vi "DC filter(Sub VI).vi"(0 "AI0 input":dbl[](array[numeric]), 1 "AI1 input":dbl[](array[numeric]), 2 "AI2 input":dbl[](array[numeric]), 3 "AI3 input":dbl[](array[numeric]), 4 "AI4 input":dbl[](array[numeric]), 5 "AI5 input":dbl[](array[numeric]), 6 "AI6 input":dbl[](array[numeric]), 7 "AI7 input":dbl[](array[numeric]), 8 "sum input (回授)":dbl[](array[numeric]), 9 "DAQ AI":dbl[](array[numeric]), 10 "迴圈數":i32, 11 "ÂoDC°}¦C¤j¤p":i32) -> (17 "sum out":dbl[](array[numeric]), 18 "DC Filter out":dbl[](array[numeric]), 19 "DC value":dbl[](array[numeric]), 20 "AI0 output":dbl[](array[numeric]), 21 "AI1 output":dbl[](array[numeric]), 22 "AI2 output":dbl[](array[numeric]), 23 "AI3 output":dbl[](array[numeric]), 24 "AI4 output":dbl[](array[numeric]), 25 "AI5 output":dbl[](array[numeric]), 26 "AI6 output":dbl[](array[numeric]), 27 "AI7 output":dbl[](array[numeric]))   [LabVIEW 2010]
panel:
  # "output"
  # "input"
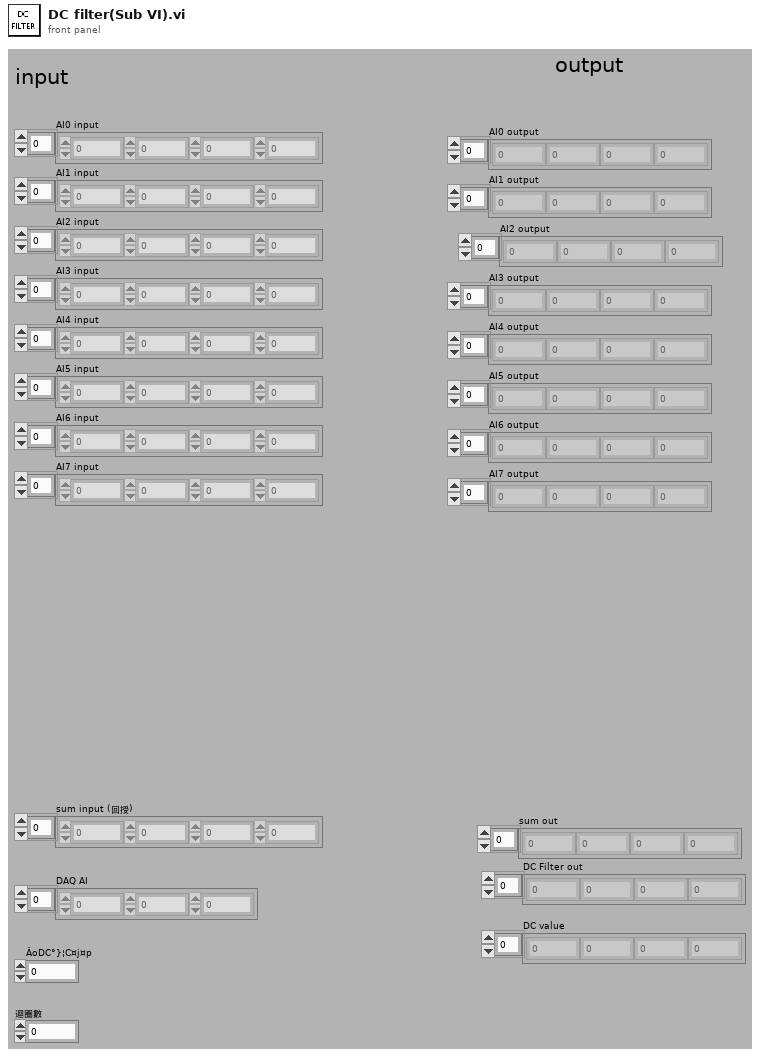
[diagram p1: front panel]
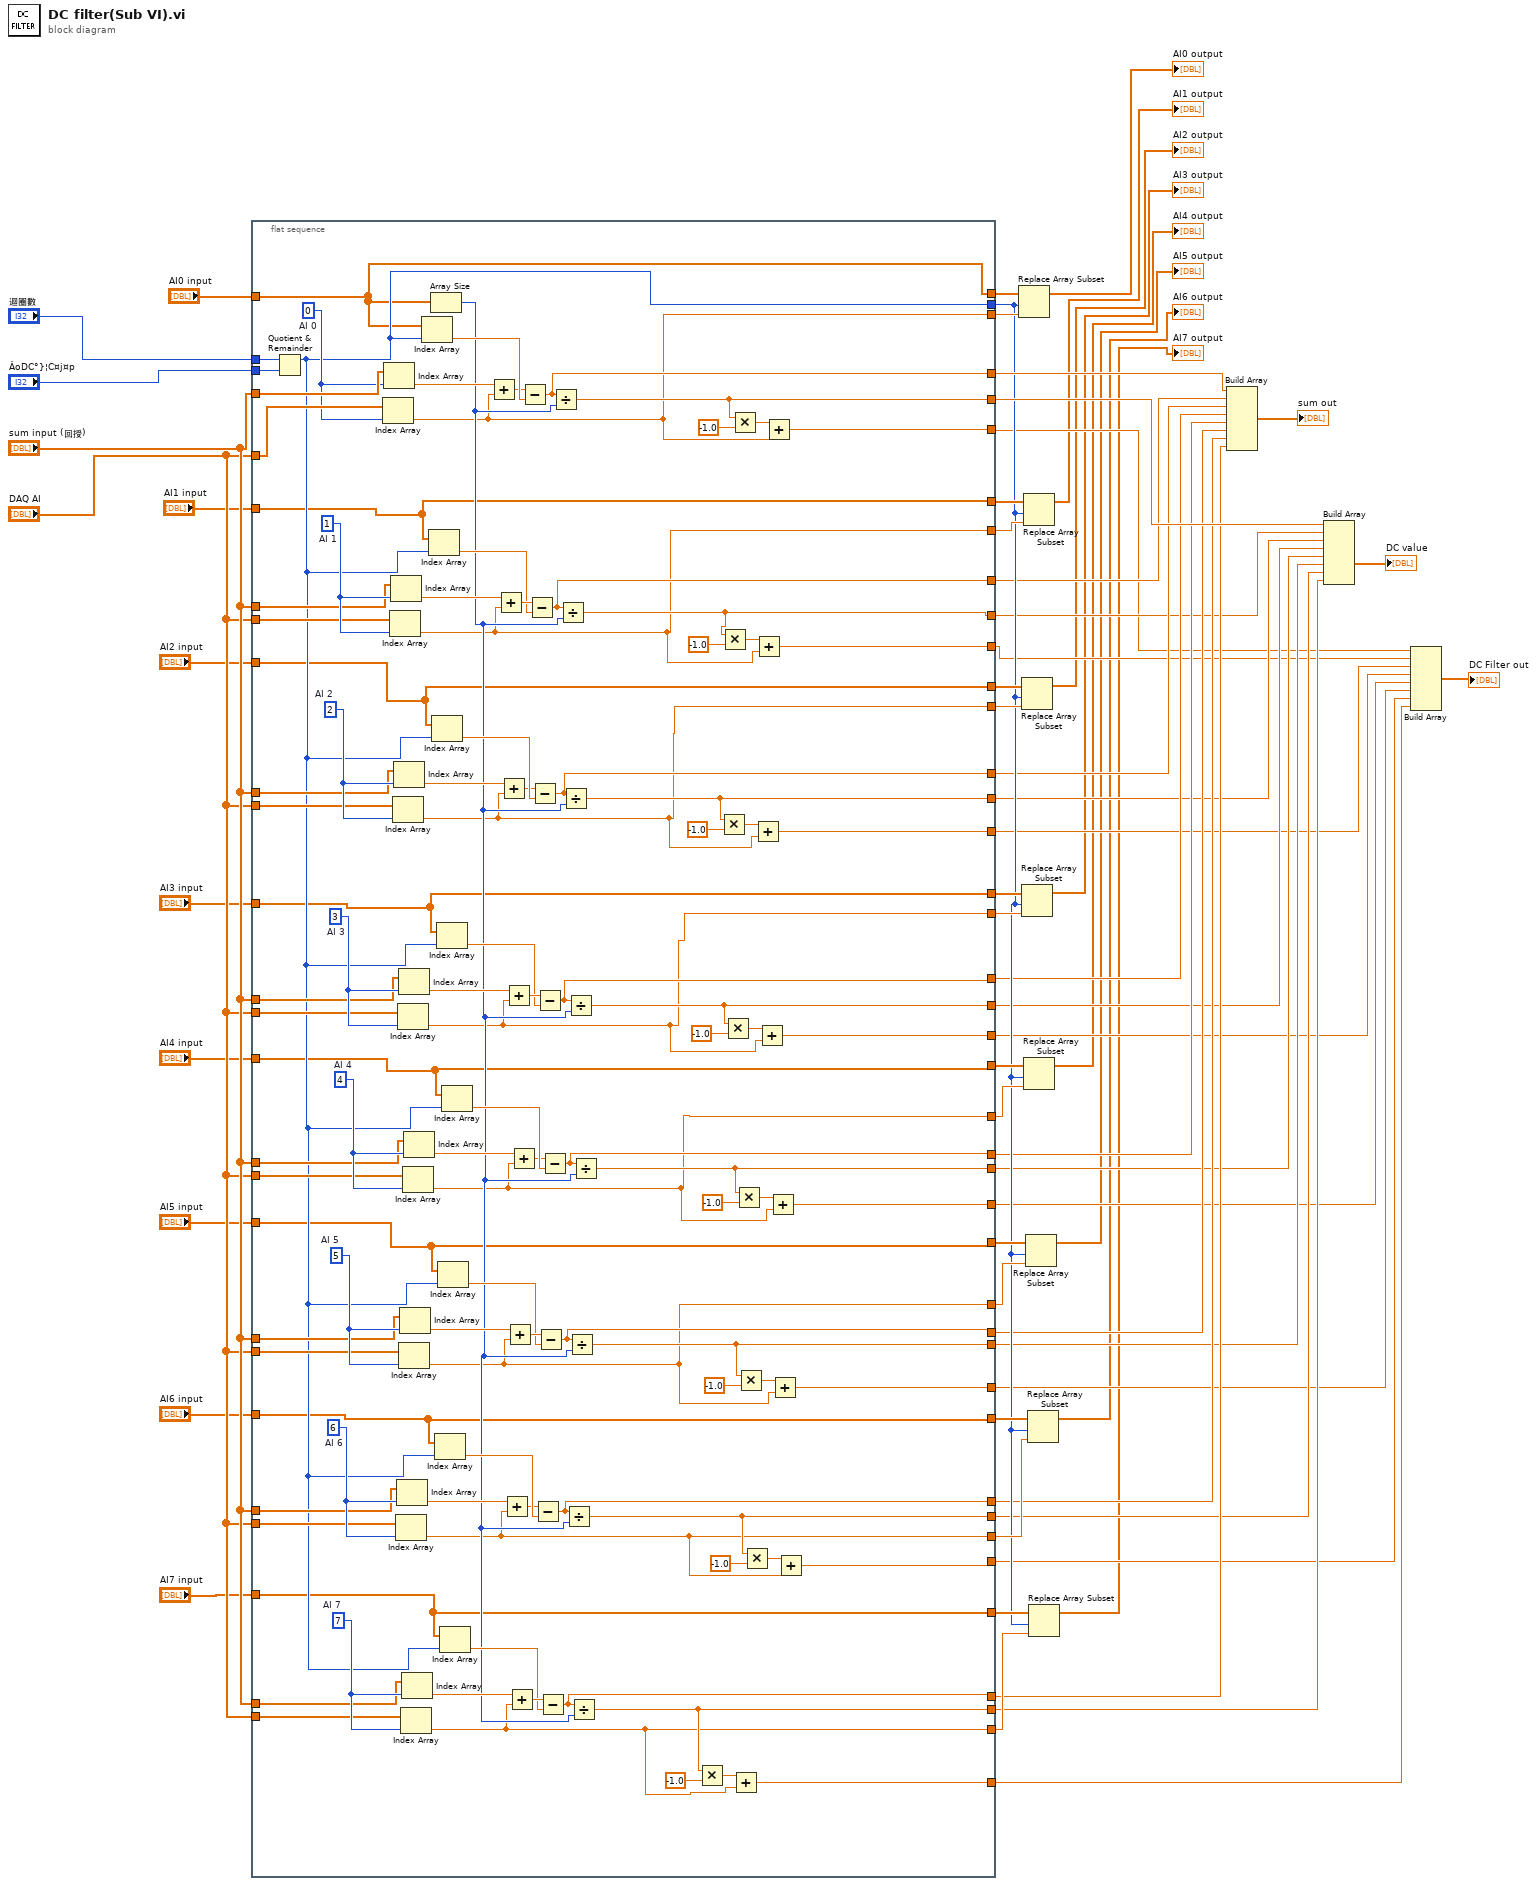
[diagram p0: block diagram]
diagram:
  n1 = flat-sequence {
    tunnel: [w109] -> w62
    tunnel: [w121] -> w42
    tunnel: [w72] -> w61
    tunnel: "迴圈數" -> [w164]
    tunnel: "sum input (回授)" -> [w169]
    tunnel: "DAQ AI" -> [w168]
    tunnel: "ÂoDC°}¦C¤j¤p" -> [w167]
    tunnel: [w112] -> w60
    tunnel: [w165] -> w63
    tunnel: "sum input (回授)" -> [w159]
    tunnel: "DAQ AI" -> [w158]
    tunnel: [w71] -> w57
    tunnel: [w105] -> w56
    tunnel: "sum input (回授)" -> [w153]
    tunnel: "DAQ AI" -> [w152]
    tunnel: [w70] -> w55
    tunnel: [w101] -> w54
    tunnel: "sum input (回授)" -> [w147]
    tunnel: "DAQ AI" -> [w146]
    tunnel: [w69] -> w53
    tunnel: [w97] -> w52
    tunnel: "sum input (回授)" -> [w129]
    tunnel: "sum input (回授)" -> [w128]
    tunnel: "sum input (回授)" -> [w127]
    tunnel: "sum input (回授)" -> [w126]
    tunnel: "DAQ AI" -> [w125]
    tunnel: "DAQ AI" -> [w124]
    tunnel: "DAQ AI" -> [w123]
    tunnel: "DAQ AI" -> [w122]
    tunnel: [w68] -> w49
    tunnel: [w93] -> w48
    tunnel: [w67] -> w47
    tunnel: [w89] -> w46
    tunnel: [w66] -> w45
    tunnel: [w85] -> w44
    tunnel: [w65] -> w43
    tunnel: [w81] -> w40
    tunnel: [w120] -> w39
    tunnel: [w119] -> w38
    tunnel: [w118] -> w37
    tunnel: [w117] -> w36
    tunnel: [w116] -> w35
    tunnel: [w115] -> w34
    tunnel: [w114] -> w33
    tunnel: [w106] -> w32
    tunnel: [w102] -> w31
    tunnel: [w98] -> w30
    tunnel: [w94] -> w29
    tunnel: [w90] -> w28
    tunnel: [w86] -> w27
    tunnel: [w82] -> w26
    tunnel: [w80] -> w17
    tunnel: [w79] -> w18
    tunnel: [w78] -> w19
    tunnel: [w77] -> w20
    tunnel: [w76] -> w21
    tunnel: [w75] -> w22
    tunnel: [w74] -> w23
    tunnel: [w73] -> w24
    tunnel: "AI0 input" -> [w72]
    tunnel: "AI1 input" -> [w71]
    tunnel: "AI2 input" -> [w70]
    tunnel: "AI3 input" -> [w69]
    tunnel: "AI4 input" -> [w68]
    tunnel: "AI5 input" -> [w67]
    tunnel: "AI6 input" -> [w66]
    tunnel: "AI7 input" -> [w65]
    frame #0 {
      w133 = 7  # AI 7
      w134 = 6  # AI 6
      w141 = 5  # AI 5
      w142 = 4  # AI 4
      w151 = 3  # AI 3
      w154 = 2  # AI 2
      w163 = 1  # AI 1
      w166 = 0  # AI 0
      n2 = Quotient & Remainder(x=w164, y=w167) -> (x-y*floor(x/y)=w121:i32)  [unwired: 1 out]
      n3 = Index Array(array=w168, index=w166) -> (element=w109:dbl)
      n4 = Index Array(array=w169, index=w166) -> (element=w170:dbl)
      n5 = Index Array(array=w158, index=w163) -> (element=w105:dbl)
      n6 = Index Array(array=w159, index=w163) -> (element=w162:dbl)
      n7 = Index Array(array=w152, index=w154) -> (element=w101:dbl)
      n8 = Index Array(array=w153, index=w154) -> (element=w155:dbl)
      n9 = Index Array(array=w123, index=w134) -> (element=w85:dbl)
      n10 = Index Array(array=w127, index=w134) -> (element=w135:dbl)
      n11 = Index Array(array=w146, index=w151) -> (element=w97:dbl)
      n12 = Index Array(array=w147, index=w151) -> (element=w150:dbl)
      n13 = Index Array(array=w124, index=w141) -> (element=w89:dbl)
      n14 = Index Array(array=w128, index=w141) -> (element=w140:dbl)
      n15 = Index Array(array=w122, index=w133) -> (element=w81:dbl)
      n16 = Index Array(array=w126, index=w133) -> (element=w132:dbl)
      n17 = Index Array(array=w125, index=w142) -> (element=w93:dbl)
      n18 = Index Array(array=w129, index=w142) -> (element=w143:dbl)
      n19 = Index Array(array=w72, index=w121) -> (element=w172:dbl)
      n20 = Index Array(array=w71, index=w121) -> (element=w160:dbl)
      n21 = Array Size(array=w72) -> (size(s)=w113:i32)
      n22 = Index Array(array=w70, index=w121) -> (element=w157:dbl)
      n23 = Index Array(array=w66, index=w121) -> (element=w137:dbl)
      n24 = Index Array(array=w69, index=w121) -> (element=w148:dbl)
      n25 = Index Array(array=w67, index=w121) -> (element=w138:dbl)
      n26 = Index Array(array=w65, index=w121) -> (element=w130:dbl)
      n27 = Index Array(array=w68, index=w121) -> (element=w145:dbl)
      n28 = Add(x=w170, y=w109) -> (x+y=w171:dbl)
      n29 = Add(x=w162, y=w105) -> (x+y=w161:dbl)
      n30 = Add(x=w155, y=w101) -> (x+y=w156:dbl)
      n31 = Add(x=w135, y=w85) -> (x+y=w136:dbl)
      n32 = Add(x=w150, y=w97) -> (x+y=w149:dbl)
      n33 = Add(x=w140, y=w89) -> (x+y=w139:dbl)
      n34 = Add(x=w132, y=w81) -> (x+y=w131:dbl)
      n35 = Add(x=w143, y=w93) -> (x+y=w144:dbl)
      n36 = Subtract(x=w171, y=w172) -> (x-y=w165:dbl)
      n37 = Subtract(x=w161, y=w160) -> (x-y=w120:dbl)
      n38 = Subtract(x=w156, y=w157) -> (x-y=w119:dbl)
      n39 = Subtract(x=w136, y=w137) -> (x-y=w115:dbl)
      n40 = Subtract(x=w149, y=w148) -> (x-y=w118:dbl)
      n41 = Subtract(x=w139, y=w138) -> (x-y=w116:dbl)
      n42 = Subtract(x=w131, y=w130) -> (x-y=w114:dbl)
      n43 = Subtract(x=w144, y=w145) -> (x-y=w117:dbl)
      n44 = Divide(x=w165, y=w113) -> (x/y=w112:dbl)
      n45 = Divide(x=w120, y=w113) -> (x/y=w106:dbl)
      n46 = Divide(x=w119, y=w113) -> (x/y=w102:dbl)
      n47 = Divide(x=w115, y=w113) -> (x/y=w86:dbl)
      n48 = Divide(x=w118, y=w113) -> (x/y=w98:dbl)
      n49 = Divide(x=w116, y=w113) -> (x/y=w90:dbl)
      n50 = Divide(x=w114, y=w113) -> (x/y=w82:dbl)
      n51 = Divide(x=w117, y=w113) -> (x/y=w94:dbl)
      n52 = Multiply(x=w82, y=-1.0) -> (x*y=w83:dbl)
      n53 = Multiply(x=w102, y=-1.0) -> (x*y=w103:dbl)
      n54 = Multiply(x=w106, y=-1.0) -> (x*y=w107:dbl)
      n55 = Multiply(x=w98, y=-1.0) -> (x*y=w99:dbl)
      n56 = Multiply(x=w112, y=-1.0) -> (x*y=w110:dbl)
      n57 = Add(x=w83, y=w81) -> (x+y=w80:dbl)
      n58 = Multiply(x=w94, y=-1.0) -> (x*y=w95:dbl)
      n59 = Multiply(x=w90, y=-1.0) -> (x*y=w91:dbl)
      n60 = Multiply(x=w86, y=-1.0) -> (x*y=w87:dbl)
      n61 = Add(x=w103, y=w101) -> (x+y=w75:dbl)
      n62 = Add(x=w107, y=w105) -> (x+y=w74:dbl)
      n63 = Add(x=w99, y=w97) -> (x+y=w76:dbl)
      n64 = Add(x=w110, y=w109) -> (x+y=w73:dbl)
      n65 = Add(x=w95, y=w93) -> (x+y=w77:dbl)
      n66 = Add(x=w91, y=w89) -> (x+y=w78:dbl)
      n67 = Add(x=w87, y=w85) -> (x+y=w79:dbl)
    }
  }
  n68 = Replace Array Subset(array=w61, new element=w62, index=w42) -> (→"AI0 output":dbl[])
  n69 = Replace Array Subset(array=w55, new element=w54, index=w42) -> (→"AI2 output":dbl[])
  n70 = Replace Array Subset(array=w53, new element=w52, index=w42) -> (→"AI3 output":dbl[])
  n71 = Replace Array Subset(array=w57, new element=w56, index=w42) -> (→"AI1 output":dbl[])
  n72 = Replace Array Subset(array=w49, new element=w48, index=w42) -> (→"AI4 output":dbl[])
  n73 = Replace Array Subset(array=w47, new element=w46, index=w42) -> (→"AI5 output":dbl[])
  n74 = Replace Array Subset(array=w45, new element=w44, index=w42) -> (→"AI6 output":dbl[])
  n75 = Replace Array Subset(array=w43, new element=w40, index=w42) -> (→"AI7 output":dbl[])
  n76 = Build Array(w63, w39, w38, w37, w36, w35, w34, w33) -> (→"sum out":dbl[])
  n77 = Build Array(w60, w32, w31, w30, w29, w28, w27, w26) -> (→"DC value":dbl[])
  n78 = Build Array(w24, w23, w22, w21, w20, w19, w18, w17) -> (→"DC Filter out":dbl[])
